vi "Create.vi"() -> (3 "AF Queue Stream out":refnum<class "AF Queue Stream.lvclass">)   [LabVIEW 2020, in "AF Queue Stream.lvclass"]
uses:
  AF Queue Stream.lvclass
  <vilib>/ActorFramework/Message Queue/Message Queue.lvclass
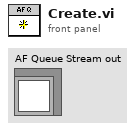
[diagram p1: front panel]
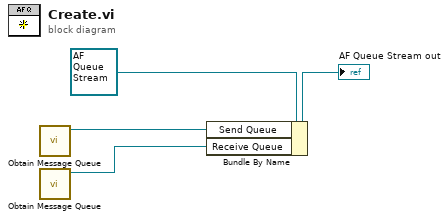
[diagram p0: block diagram]
diagram:
  n1 = call <vilib>:"Obtain Message Queue.vi"() -> ("Message Queue"=w2:refnum<class "Message Queue.lvclass">)  [unwired: 10 in, 1 out]
  n2 = call <vilib>:"Obtain Message Queue.vi"() -> ("Message Queue"=w1:refnum<class "Message Queue.lvclass">)  [unwired: 10 in, 1 out]
  n3 = Bundle By Name(cluster=refnum<class "AF Queue Stream.lvclass"> refnum ("AF Queue Stream in"), "Send Queue"=w2, "Receive Queue"=w1) -> (→"AF Queue Stream out":refnum<class "AF Queue Stream.lvclass">)
